vi "Test Failing Dummy Method.vi"(8 "error in (no error)":errorcluster, 11 "Dummy Test Case in":refnum<class "Dummy.lvclass">) -> (0 "error out":errorcluster, 3 "Dummy Test Case out":refnum<class "Dummy.lvclass">)   [LabVIEW 2020, in "Test Finder Test Dummy.lvlib" / "Dummy.lvclass"]
uses:
  Dummy.lvclass
  Dummy.lvclass/Dummy.ctl
  Core/LUnit Test Case/LUnit Test Case.lvclass
  C:/git/astemes-lunit/source/Core/LUnit Test Case/LUnit Test Case.lvclass
  C:/git/astemes-lunit/source/Core/Runnable/Runnable.lvclass
  C:/git/astemes-lunit/source/Tests/Test Finder Test/Dummy.lvclass
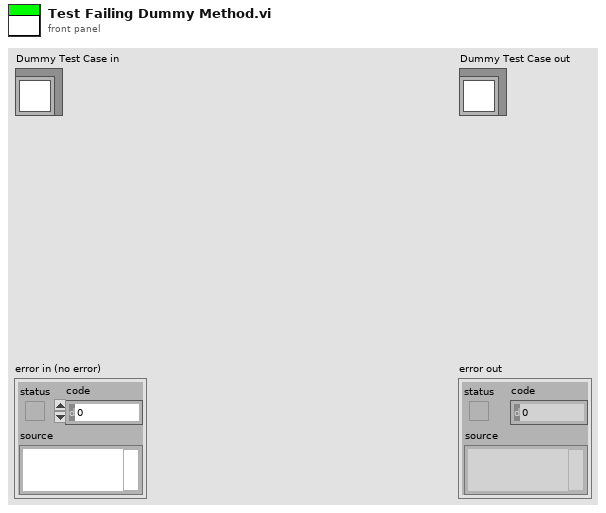
[diagram p1: front panel]
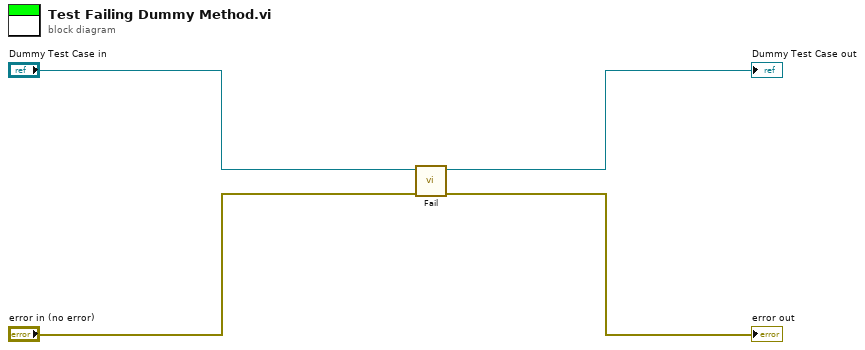
[diagram p0: block diagram]
diagram:
  n1 = call "Fail.vi"("error in (no error)"="error in (no error)", "LUnit Test Case In"="Dummy Test Case in") -> ("error out"=→"error out":errorcluster, "LUnit Test Case Out"=→"Dummy Test Case out":refnum<class "Dummy.lvclass">)  [unwired: 8 in]
